vi "Test Reply Messaging.vi"() -> ()   [LabVIEW 2020, in "Messaging Tests.lvlib" / "Messaging Tests.lvclass"]
uses:
  Messaging Tests.lvclass
  Messaging Tests.lvclass/Messaging Tests.ctl
  C:/Program Files/National Instruments/LabVIEW 2025/vi.lib/Astemes/LUnit/Test Case.lvclass
  C:/Program Files/National Instruments/LabVIEW 2025/vi.lib/Astemes/LUnit/LUnit Runnable.lvclass
  C:/dev/actor-framework/dist/Test/Unit Tests/Core/Messaging Tests/Messaging Tests/Messaging Tests.lvclass
  TestActor/Test Actor/TestActor.lvclass
  C:/dev/actor-framework/dist/vi.lib/ActorFramework/Actor/Actor.lvclass
  C:/dev/actor-framework/dist/Test/Unit Tests/Core/Messaging Tests/TestActor/Test Actor/TestActor.lvclass
  vi.lib/ActorFramework/Specialty Messages/Reply Msg/Reply Msg.lvclass
  C:/dev/actor-framework/dist/vi.lib/ActorFramework/Message/Message.lvclass
  C:/dev/actor-framework/dist/vi.lib/ActorFramework/Specialty Messages/Reply Msg/Reply Msg.lvclass
  vi.lib/ActorFramework/Actor/Actor.lvclass
  vi.lib/ActorFramework/Stop Msg/Stop Msg.lvclass
  vi.lib/ActorFramework/LastAck/Last Ack.lvclass
  TestActor/Divide Msg/Divide Msg.lvclass
  vi.lib/ActorFramework/Message Queue/Message Queue.lvclass
  vi.lib/ActorFramework/Message Dequeuer/Message Dequeuer.lvclass
  TestActor/Increment Msg/Increment Msg.lvclass
  f0a439e9-38a6-40e0-a81e-095c7712fe71.vi
  <vilib>/Astemes/LUnit/Test Case.lvclass
  4e3e2924-ebe0-4223-8dd8-0284e1a143a6.vi
  a517c490-f8bd-4132-9ecb-63c61c3529a7.vi
panel:
  out "Test Case Out":refnum<class "Messaging Tests.lvclass">
  in  "Test Case In":refnum<class "Messaging Tests.lvclass">
  out "error out":errorcluster
  in  "error in":errorcluster
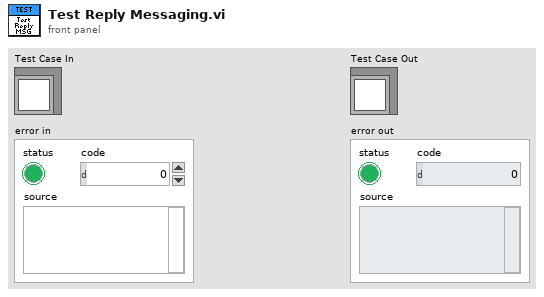
[diagram p1: front panel]
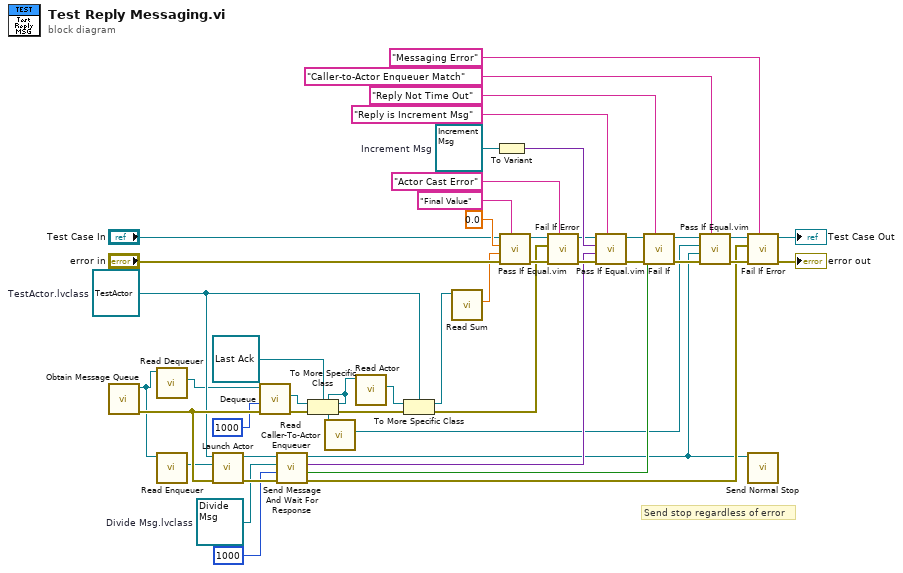
[diagram p0: block diagram]
diagram:
  w24 = refnum<class "Increment Msg.lvclass"> refnum  # Increment Msg
  w23 = refnum<class "Divide Msg.lvclass"> refnum  # Divide Msg.lvclass
  w33 = refnum<class "TestActor.lvclass"> refnum  # TestActor.lvclass
  # "Send stop regardless of error"
  n1 = call "Obtain Message Queue.vi"() -> ("error out"=w47:errorcluster, "Message Queue"=w29:refnum<class "Message Queue.lvclass">)  [unwired: 10 in]
  n2 = call "Read Dequeuer.vi"("Message Queue"=w29) -> ("Message Dequeuer"=w27:refnum<class "Message Dequeuer.lvclass">)  [unwired: 10 in]
  n3 = call "Read Enqueuer.vi"("Message Queue"=w29) -> ("Message Enqueuer"=w28:refnum<class "Message Enqueuer.lvclass">)  [unwired: 10 in]
  n4 = call "Launch Actor.vi"("error in (no error)"=w47, "Actor-to-Caller Enqueuer"=w28, "Actor"=w33) -> ("error out"=w45:errorcluster, "Caller-To-Actor Enqueuer"=w22:refnum<class "Message Enqueuer.lvclass">)  [unwired: 7 in]
  n5 = call "Dequeue.vi"("error in (no error)"=w47, "timeout in ms (-1)"=1000, "Message Dequeuer in"=w27) -> ("error out"=w44:errorcluster, "Message"=w26:refnum<class "Message.lvclass">)  [unwired: 4 in, 3 out]
  n6 = call "Send Message And Wait For Response.vi"("error in (no error)"=w45, "timeout in ms (-1)"=1000, "Original Message"=w23, "Message Enqueuer in"=w22) -> ("error out"=w35:errorcluster, "timed out?"=w9:bool, "Reply"=w6:variant, "Message Enqueuer out"=w4:refnum<class "Message Enqueuer.lvclass">)  [unwired: 4 in]
  n7 = To More Specific Class(target class=refnum<class "Last Ack.lvclass"> refnum ("Actor Framework.lvlib:Last Ack"), reference=w26, error in=w44) -> (specific class reference=w25:refnum<class "Last Ack.lvclass">, error out=w46:errorcluster)
  n8 = call "Read Caller-To-Actor Enqueuer.vi"("Last Ack"=w25) -> ("Caller-to-Actor Enqueuer"=w5:refnum<class "Message Enqueuer.lvclass">)  [unwired: 10 in]
  n9 = call "Read Actor.vi"("Last Ack"=w25) -> ("Actor"=w31:refnum<class "Actor.lvclass">)  [unwired: 10 in]
  n10 = To More Specific Class(target class=w33, reference=w31, error in=w46) -> (specific class reference=w30:refnum<class "TestActor.lvclass">, error out=w40:errorcluster)
  n11 = call "Read Sum.vi"("TestActor in"=w30) -> ("Sum"=w18:dbl)  [unwired: 9 in, 1 out]
  n12 = To Variant(anything=w24) -> (Variant=w34:variant)
  n13 = call "Pass If Equal.vim"("Description"="Final Value", "error in (no error)"="error in", "Actual"=w18, "Expected"=0.0 ("x"), "LUnit Test Case In"="Test Case In") -> ("error out"=w42:errorcluster, "LUnit Test Case Out"=w21:refnum<class "Messaging Tests.lvclass">)  [unwired: 5 in]
  n14 = call <vilib>:"Fail If Error.vi"("Description"="Actor Cast Error", "error in (no error)"=w42, "Assert error"=w40, "LUnit Test Case In"=w21) -> ("error out"=w39:errorcluster, "LUnit Test Case Out"=w12:refnum<class "Messaging Tests.lvclass">)  [unwired: 6 in]
  n15 = call "Pass If Equal.vim"("Description"="Reply is Increment Msg", "error in (no error)"=w39, "Actual"=w6, "Expected"=w34, "LUnit Test Case In"=w12) -> ("error out"=w38:errorcluster, "LUnit Test Case Out"=w11:refnum<class "Messaging Tests.lvclass">)  [unwired: 5 in]
  n16 = call <vilib>:"Fail If.vi"("Description"="Reply Not Time Out", "error in (no error)"=w38, "Fail?"=w9, "LUnit Test Case In"=w11) -> ("error out"=w37:errorcluster, "LUnit Test Case Out"=w10:refnum<class "Messaging Tests.lvclass">)  [unwired: 6 in]
  n17 = call "Pass If Equal.vim"("Description"="Caller-to-Actor Enqueuer Match", "error in (no error)"=w37, "Actual"=w4, "Expected"=w5, "LUnit Test Case In"=w10) -> ("error out"=w41:errorcluster, "LUnit Test Case Out"=w20:refnum<class "Messaging Tests.lvclass">)  [unwired: 5 in]
  n18 = call <vilib>:"Fail If Error.vi"("Description"="Messaging Error", "error in (no error)"=w41, "Assert error"=w35, "LUnit Test Case In"=w20) -> ("error out"=→"error out":errorcluster, "LUnit Test Case Out"=→"Test Case Out":refnum<class "Messaging Tests.lvclass">)  [unwired: 6 in]
  n19 = call "Send Normal Stop.vi"("Message Enqueuer"=w4) -> ()  [unwired: 10 in, 1 out]
